vi "fft.vi"() -> ()   [LabVIEW 2013]
uses:
  <vilib>/ptbypt/Frequency Domain.llb/Real FFT PtByPt.vi
  <userlib>/_MGI/1D Array/MGI Running Average/MGI Running Average(DBL).vi
  <vilib>/Analysis/NI_AALBase.lvlib
  <vilib>/ptbypt/NI_PtbyPt.lvlib
panel:
  in  "Do Everything":bool
  out "maxima indexes":i32[](array[numeric])
  out "run ave check":bool
  out "Err Peak Cluster":dbl
  out "Err  Peak":dbl
  in  "stop":bool
  out "freqout Peak Cluster":dbl format="%#_10g"
  out "freqout Peak":dbl
  in  "Analyze FFT":bool
  out "FFT Graph":dbl[](graph)
  out "xscale multiplierNEW":dbl
  in  "#samples":i32=5000
  in  "Take FFT":bool
  out "Waveform Graph NEW":dbl[][](graph)
  in  "Ampl DC":dbl
  in  "Ampl Noise(stdev)":dbl
  in  "Ampl 4":dbl
  in  "Ampl 3":dbl
  in  "Ampl 2":dbl
  in  "Ampl 1":dbl
  in  "Freq 4":dbl
  in  "Freq 3":dbl
  in  "Freq 2":dbl
  in  "Freq 1":dbl
  in  "Active Noise":bool
  in  "Active 4":bool
  in  "Active 3":bool
  in  "Active 2":bool
  in  "Active 1":bool
  in  "Active DC":bool
  in  "fs":i32=10000
  in  "Build Waveform":bool
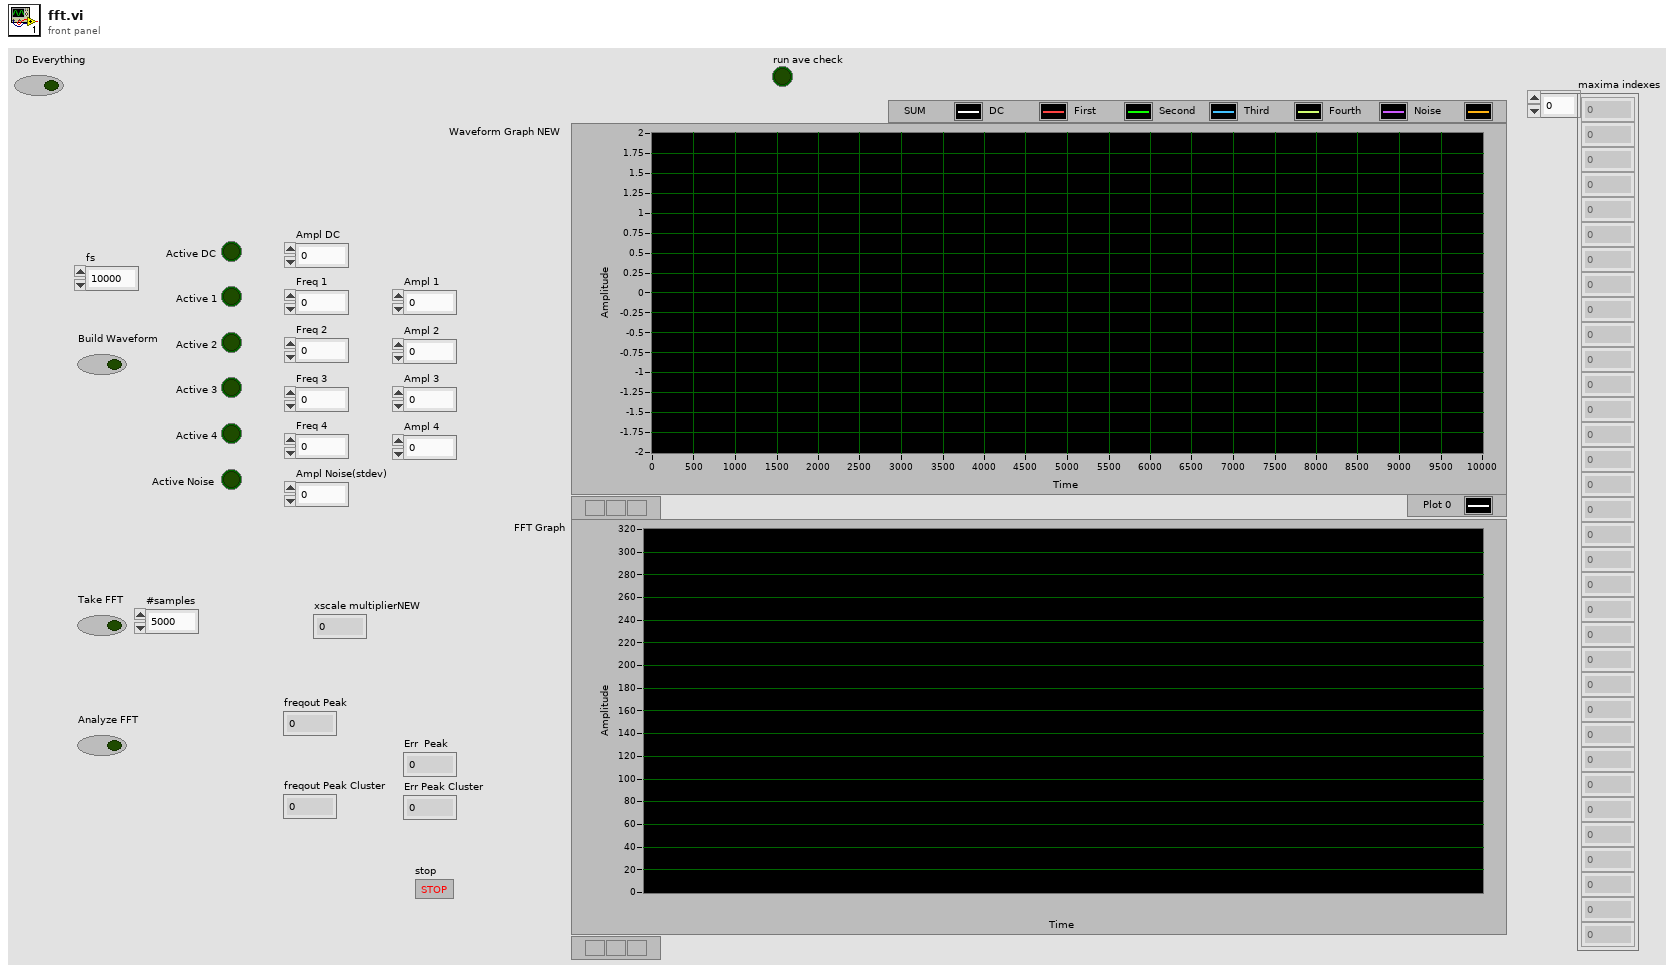
[diagram p1: front panel]
types:
  T1 = enum8{"Enabled", "Disabled", "Disabled and Grayed Out"}
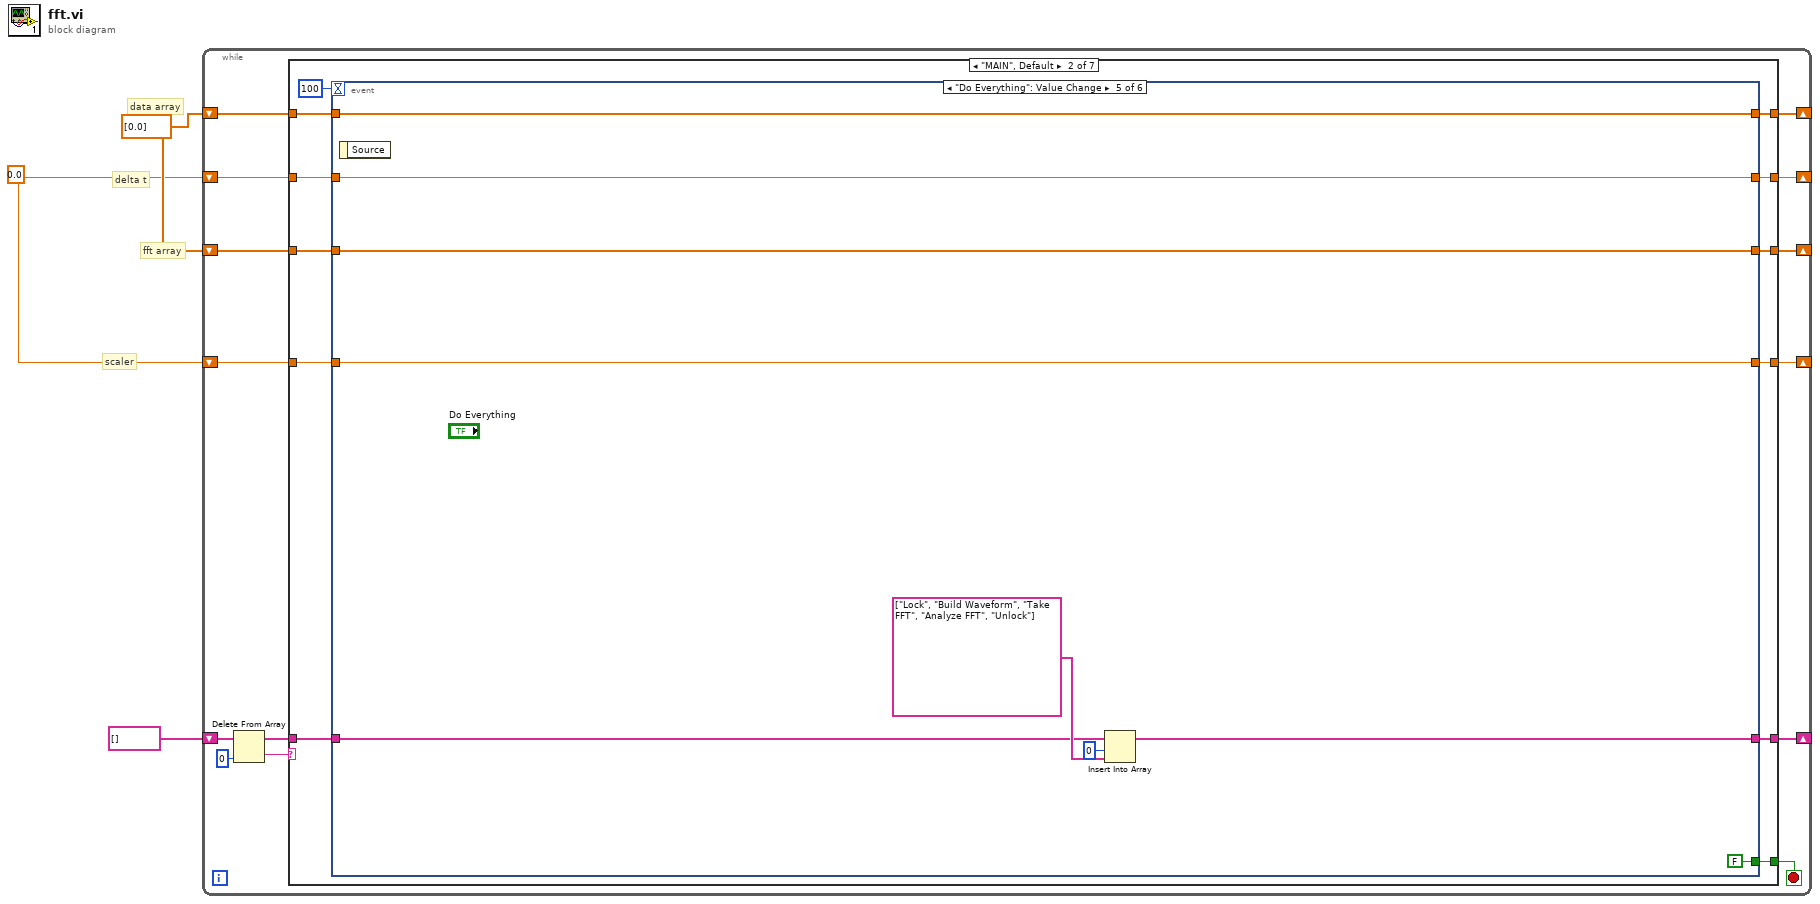
[diagram p0: block diagram]
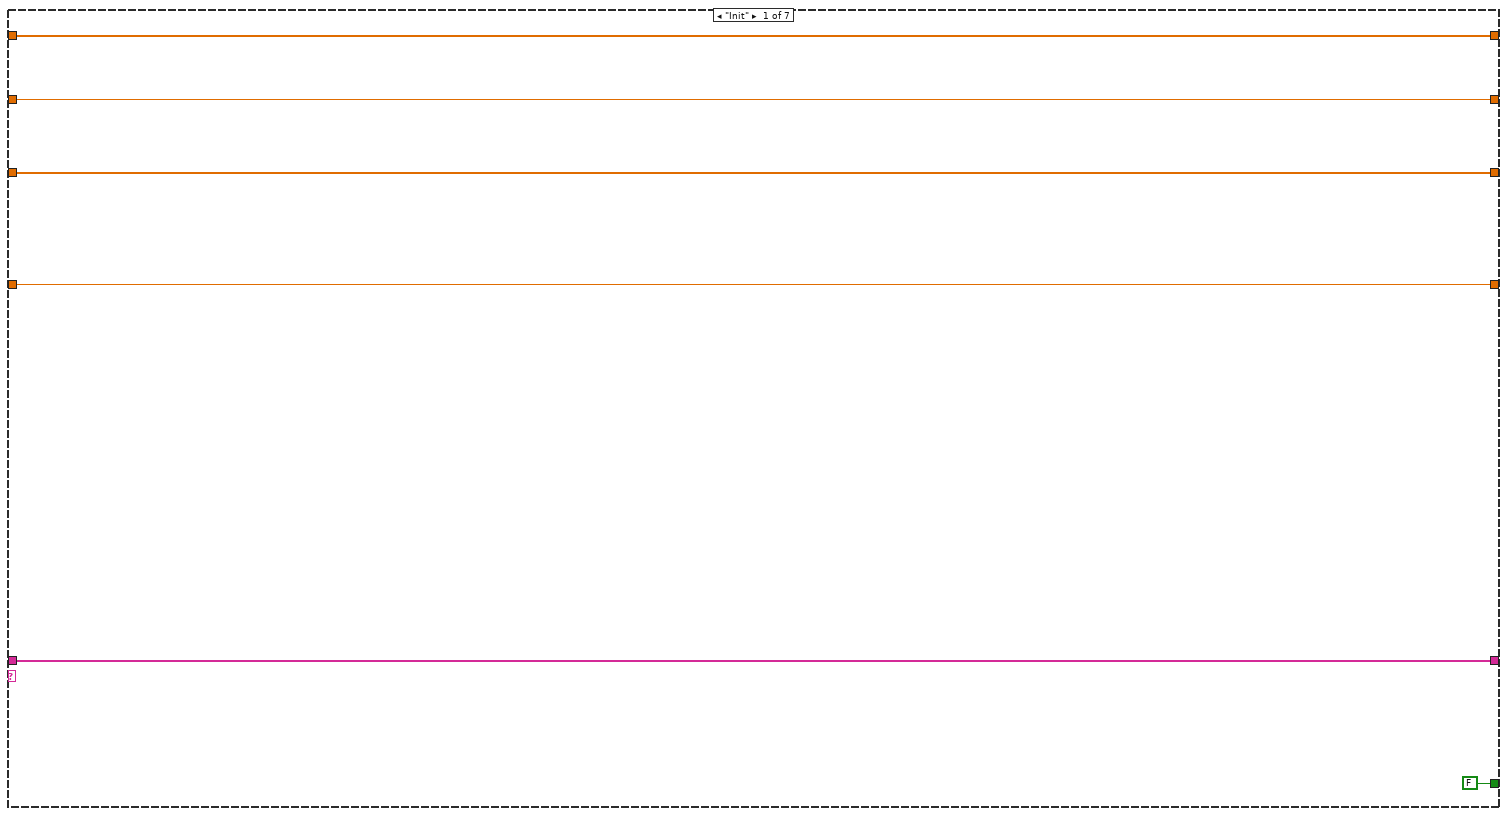
[diagram p2: hidden frame]
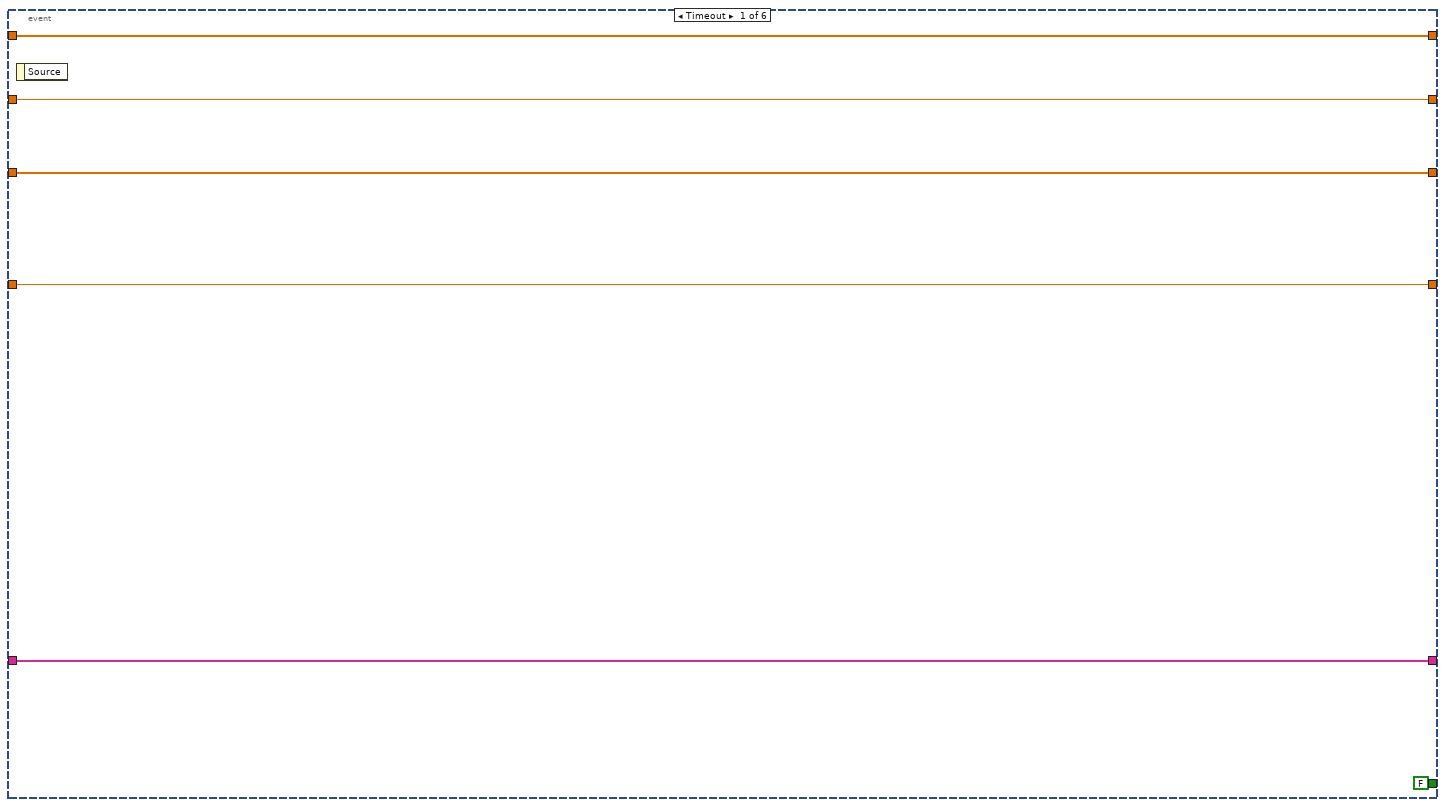
[diagram p3: hidden frame]
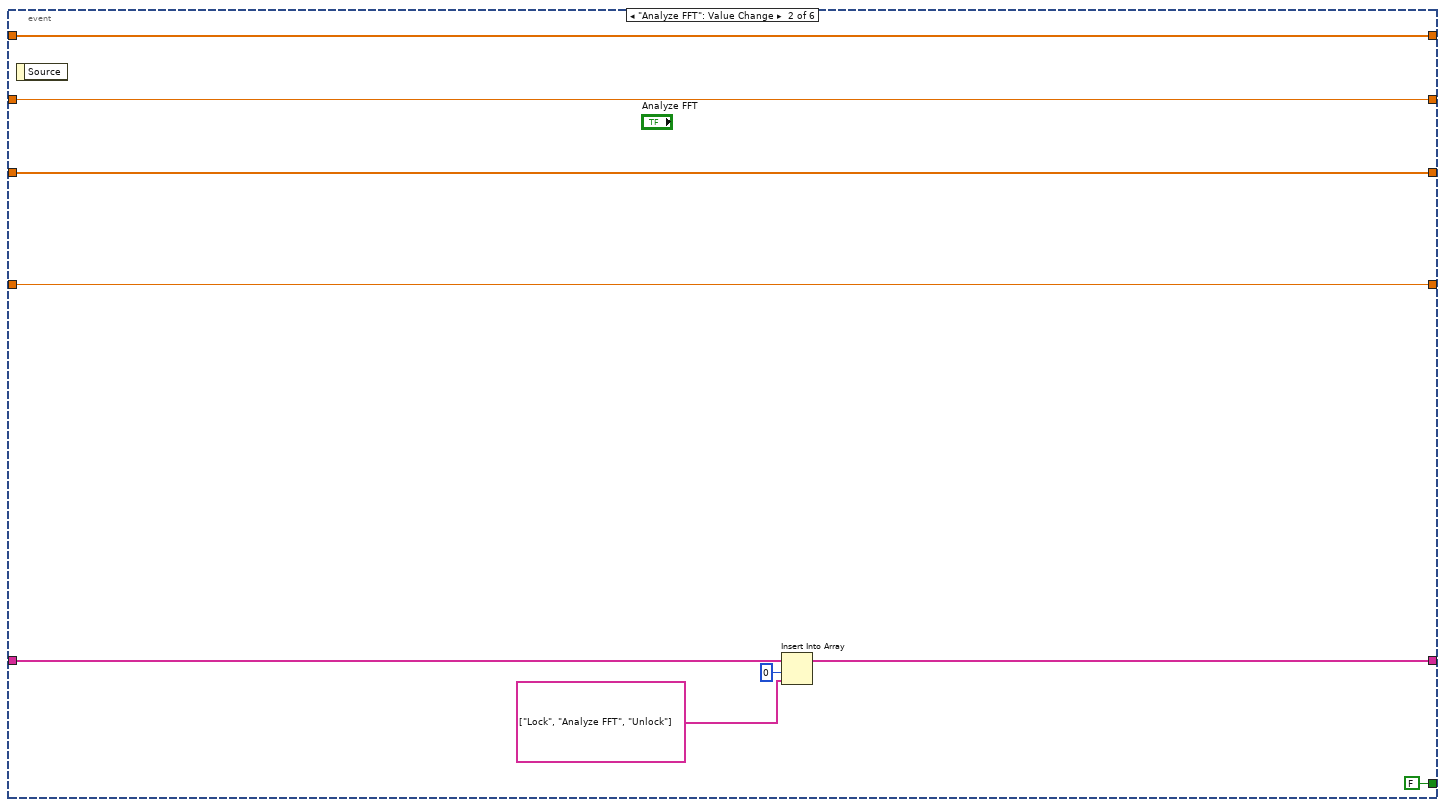
[diagram p4: hidden frame]
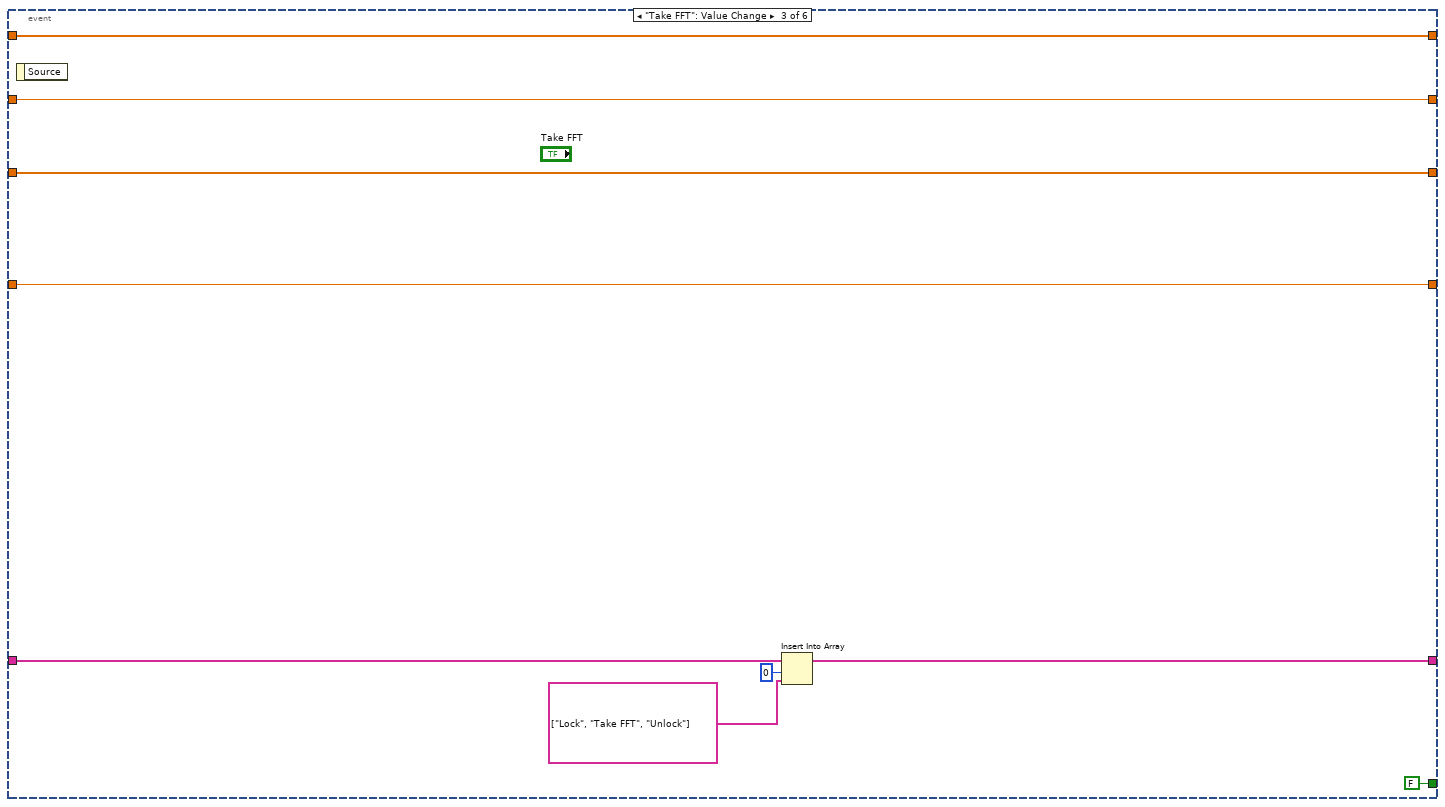
[diagram p5: hidden frame]
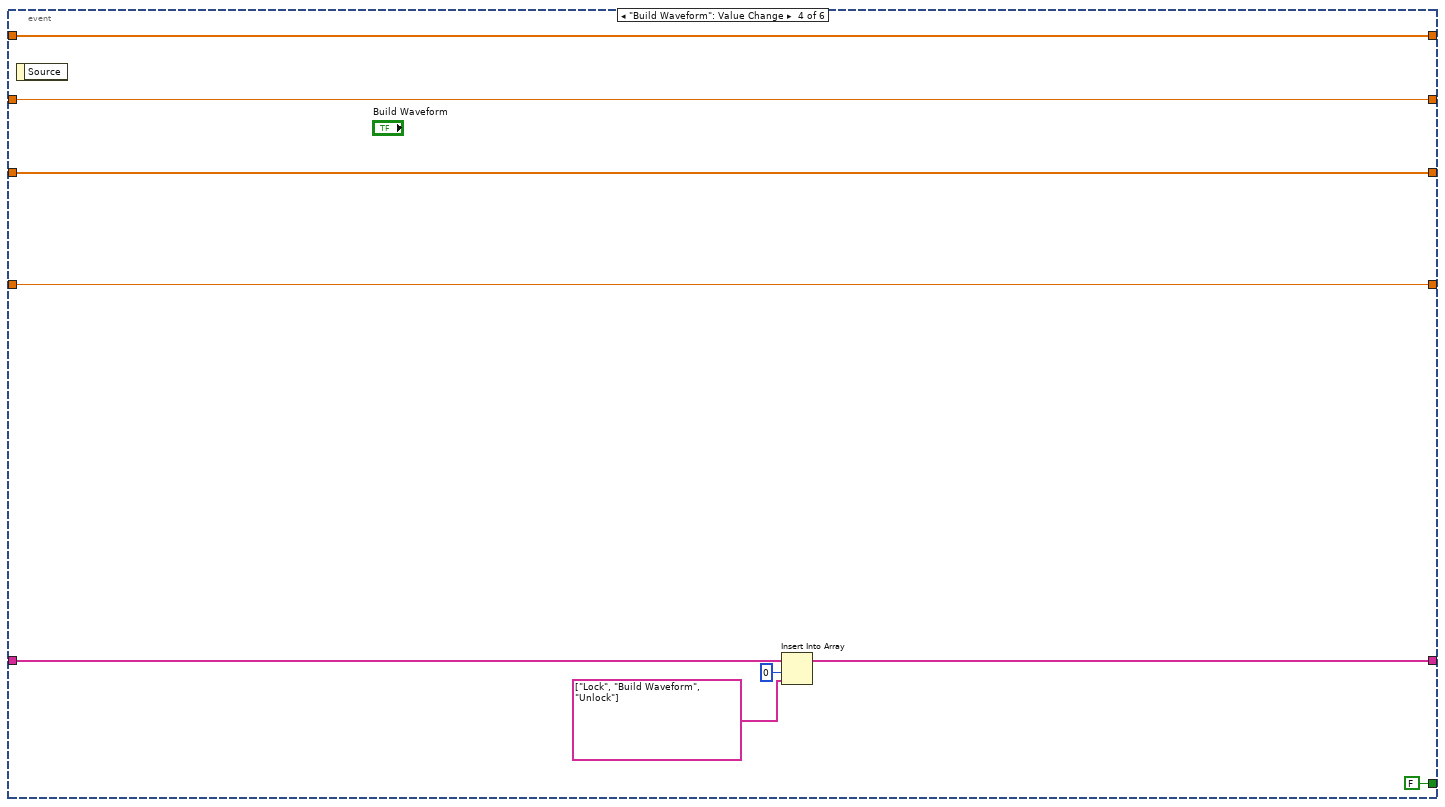
[diagram p6: hidden frame]
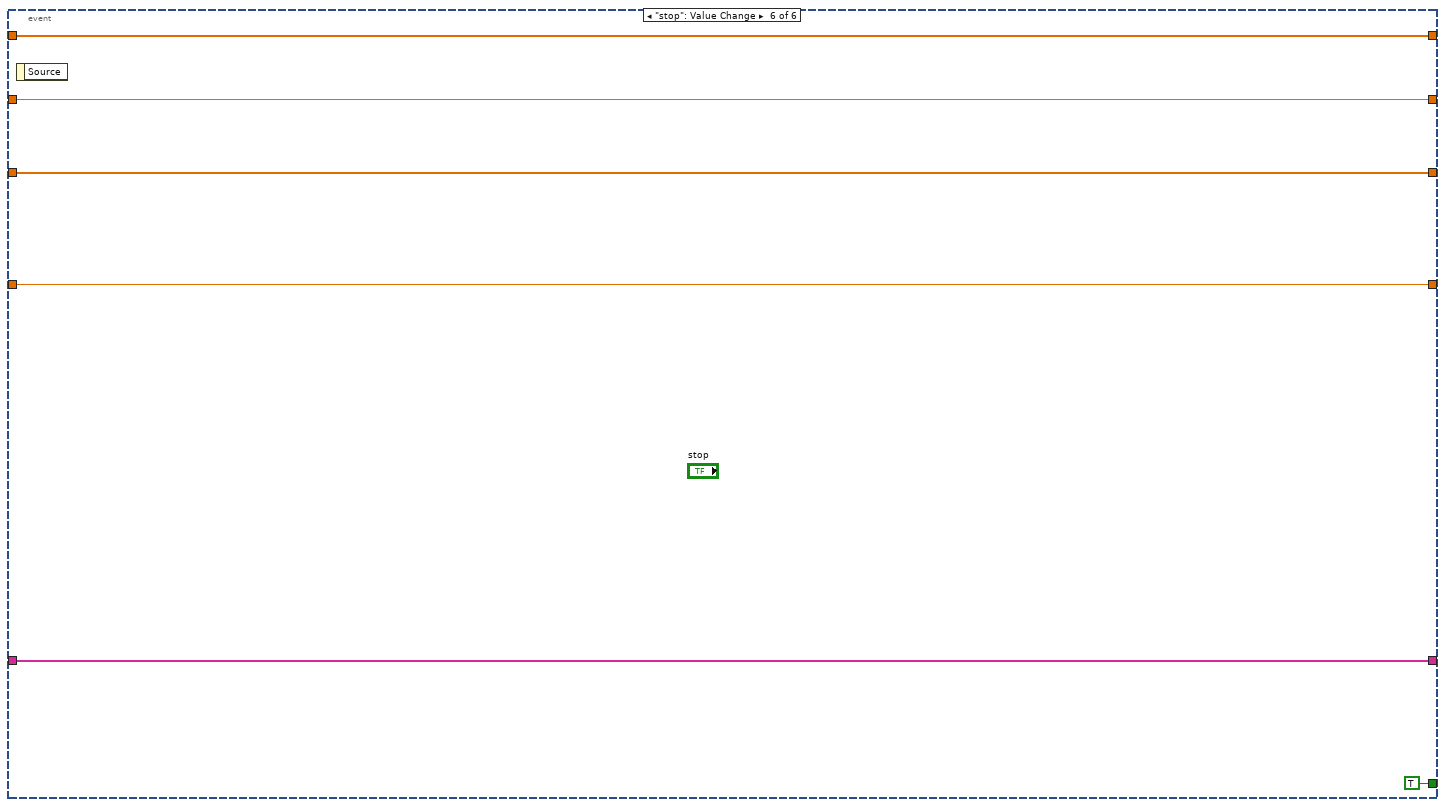
[diagram p7: hidden frame]
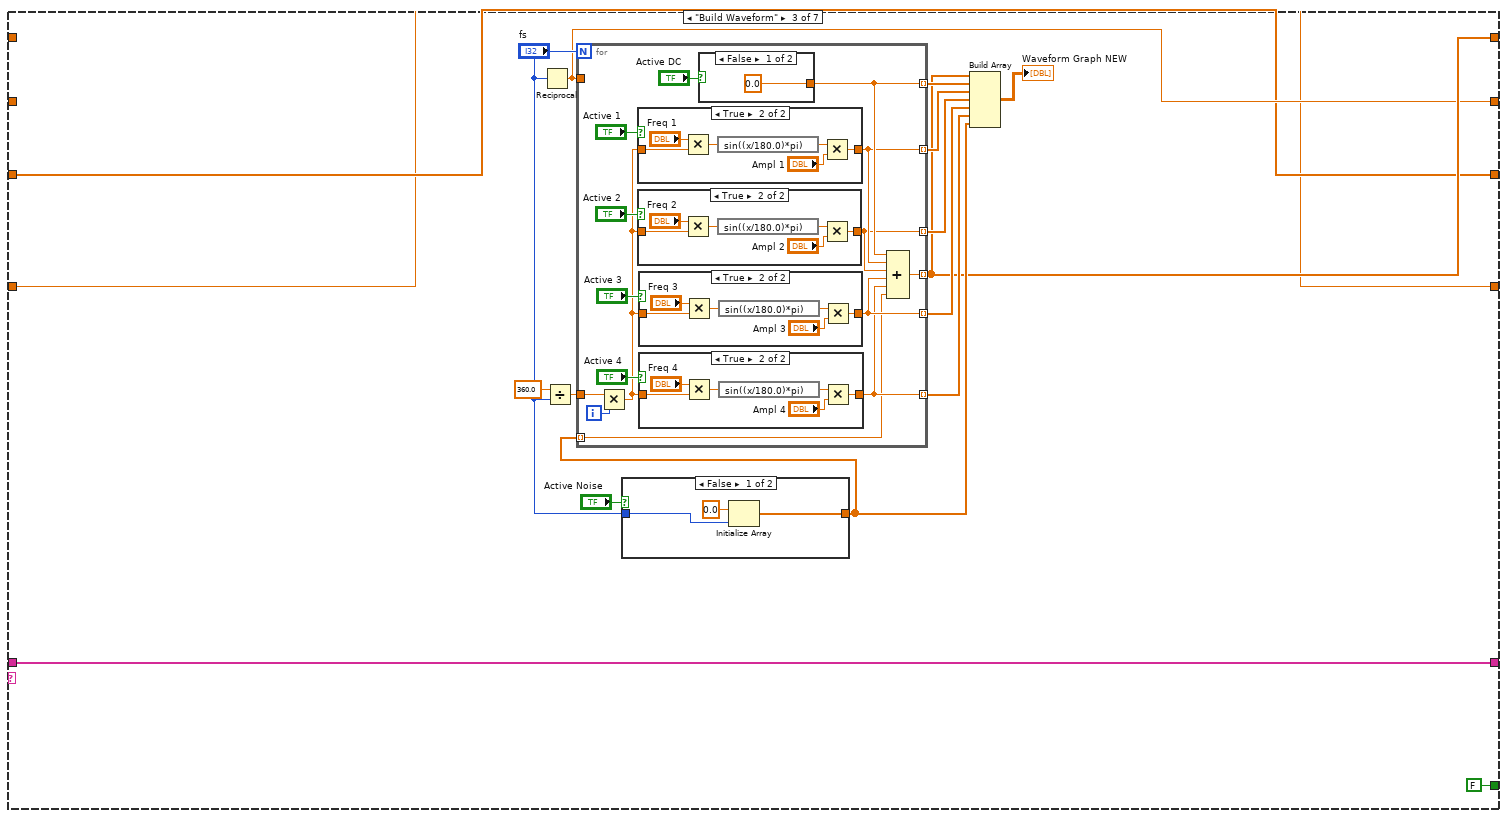
[diagram p8: hidden frame]
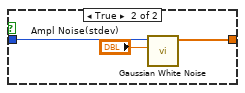
[diagram p9: hidden frame]
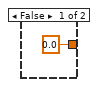
[diagram p10: hidden frame]
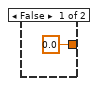
[diagram p11: hidden frame]
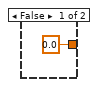
[diagram p12: hidden frame]
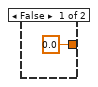
[diagram p13: hidden frame]
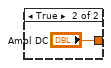
[diagram p14: hidden frame]
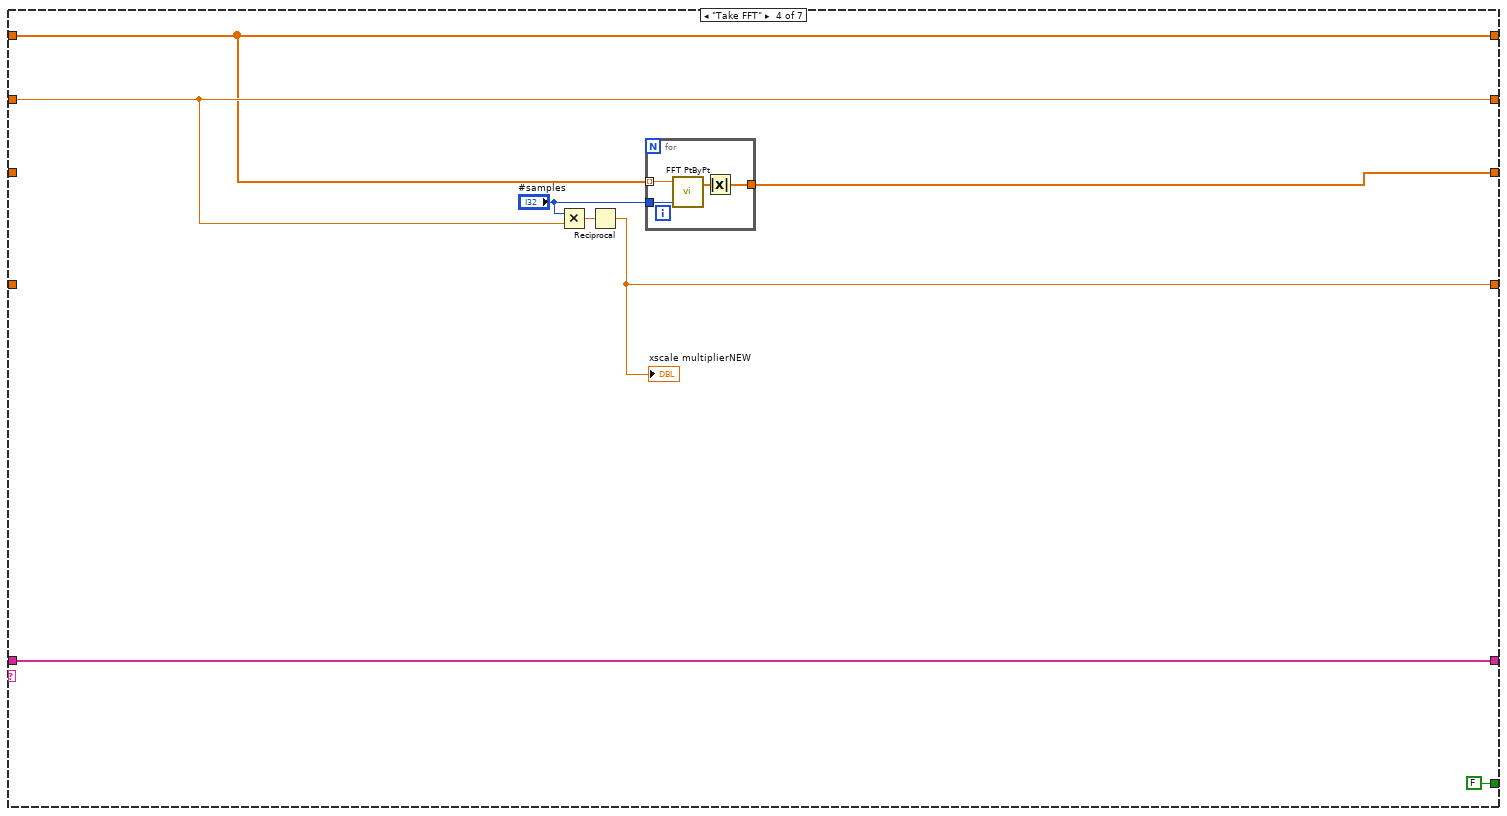
[diagram p15: hidden frame]
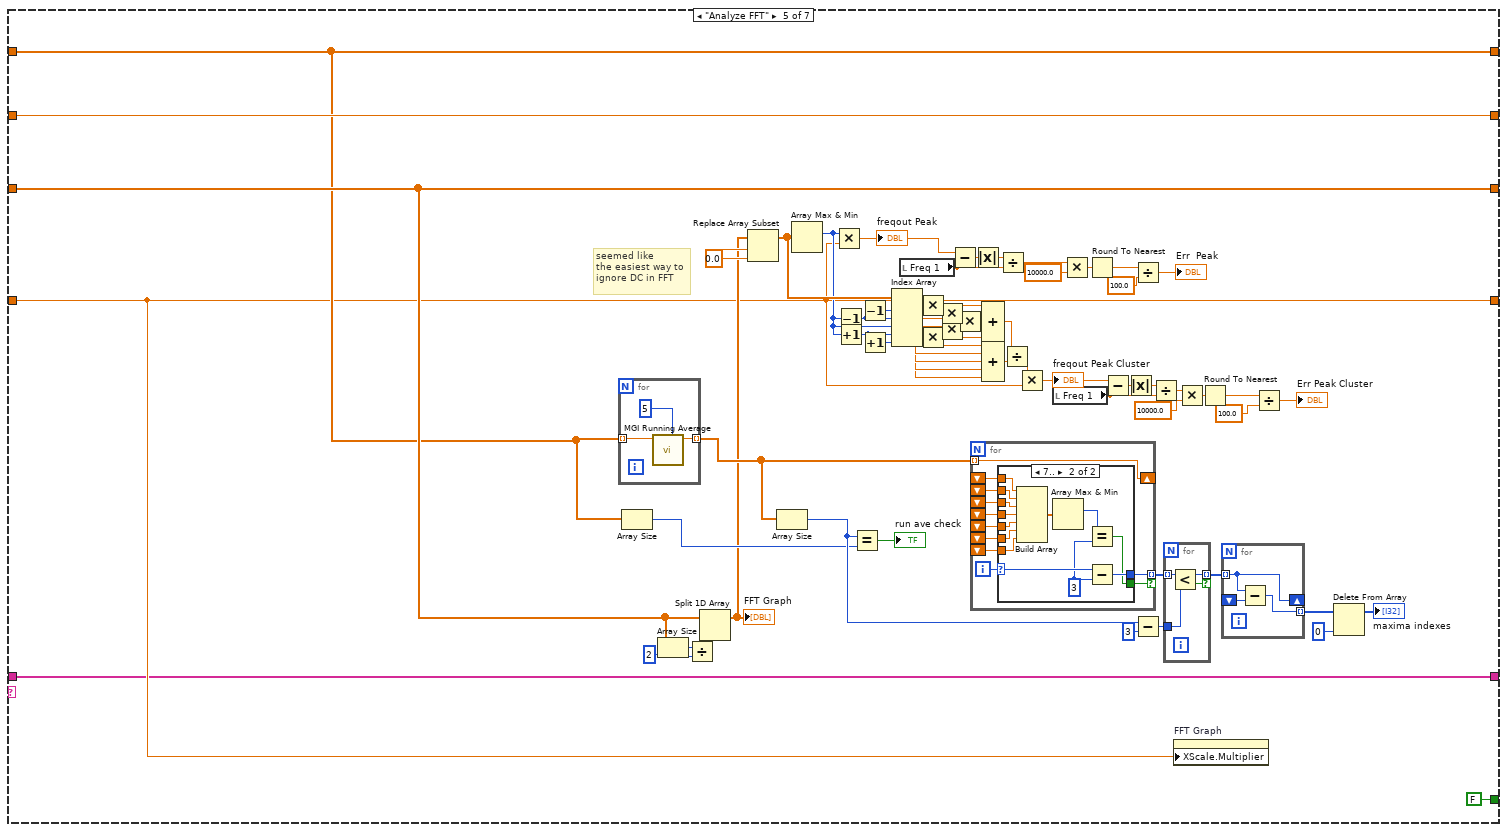
[diagram p16: hidden frame]
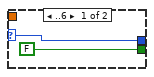
[diagram p17: hidden frame]
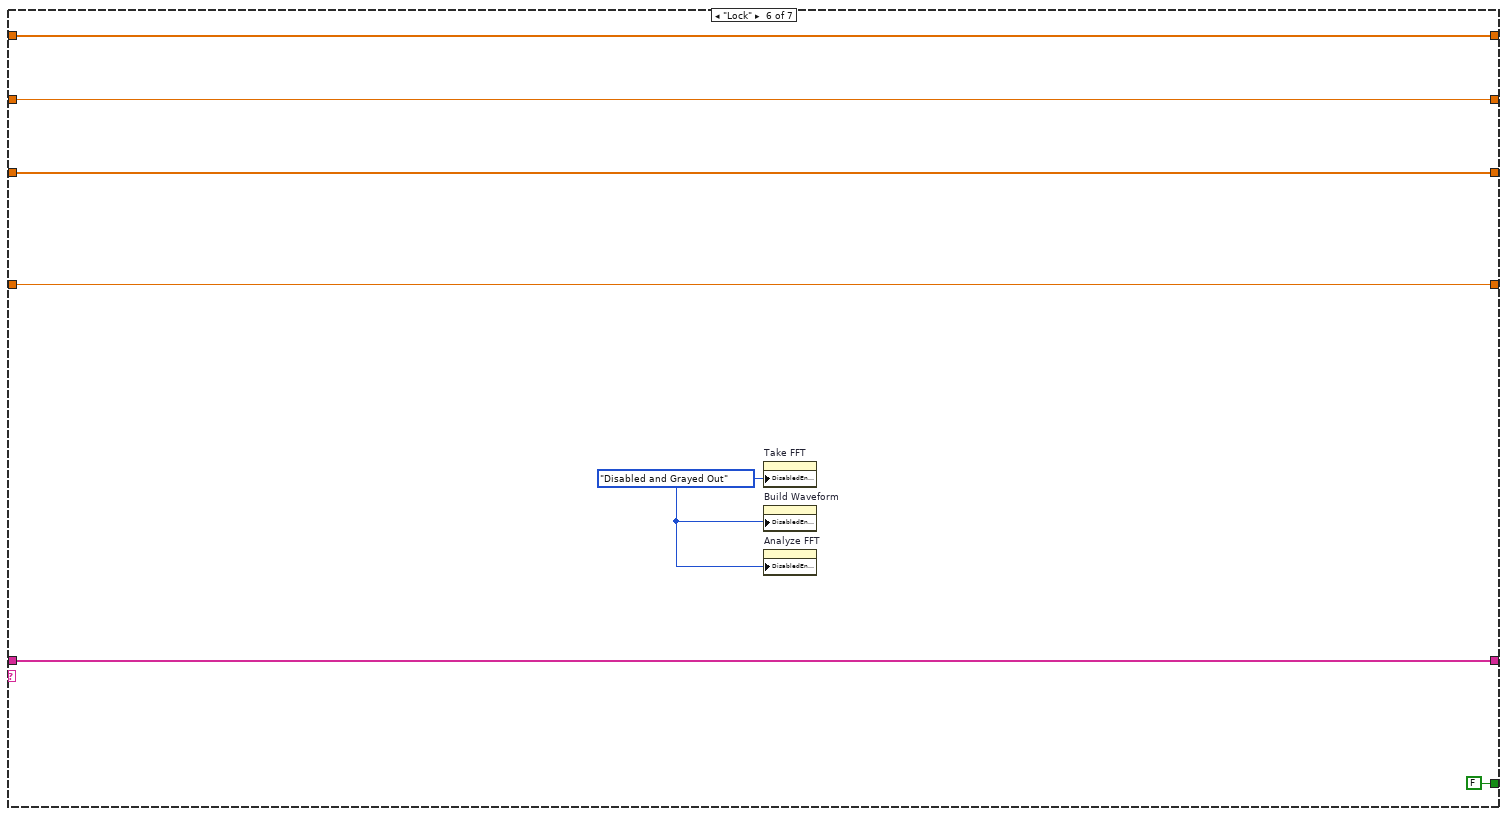
[diagram p18: hidden frame]
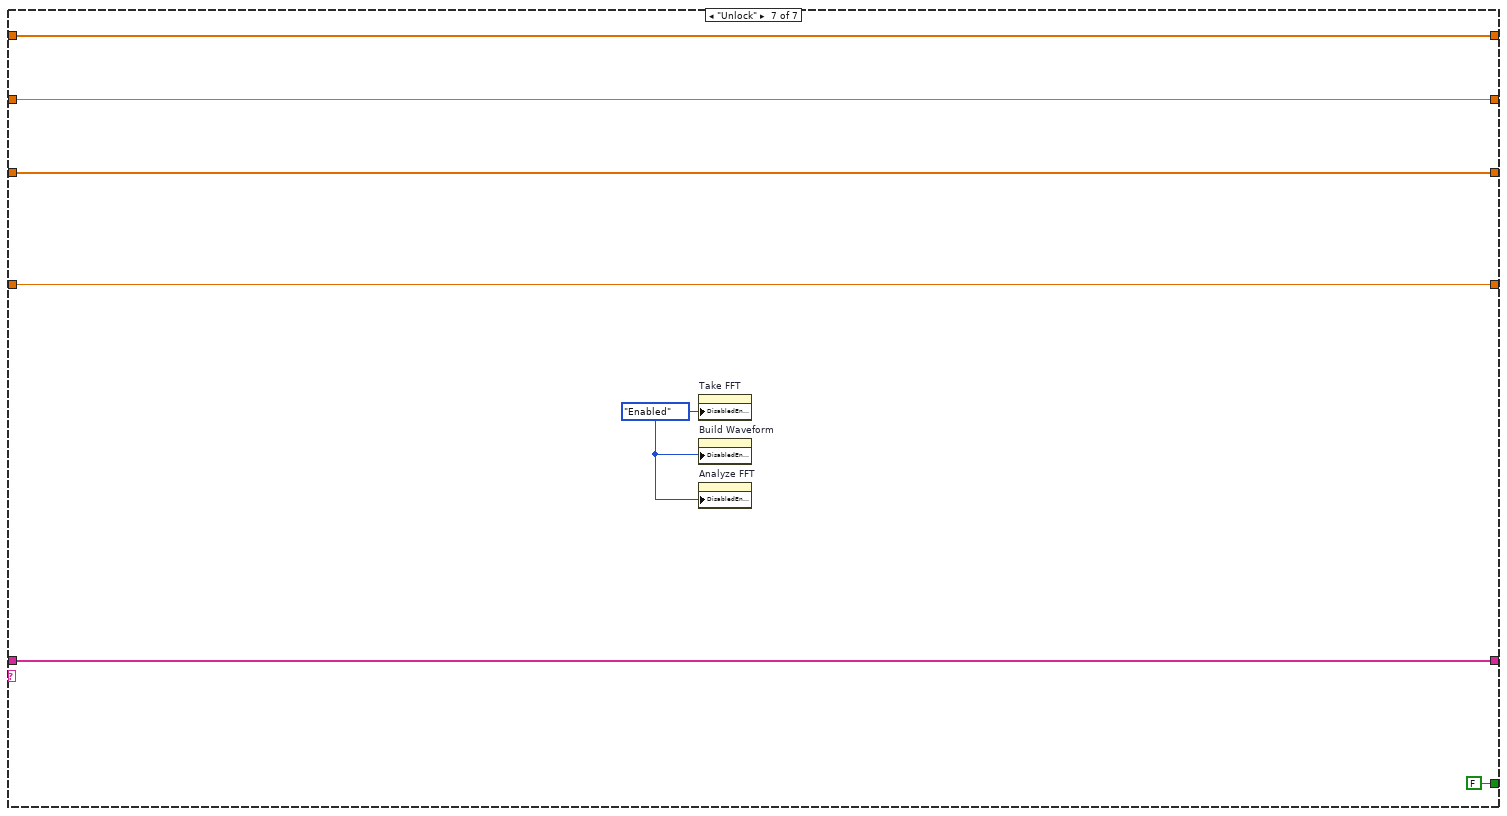
[diagram p19: hidden frame]
diagram:
  w1 = 0.0
  w2 = dbl[] [0.0]
  # "scaler"
  # "fft array"
  # "delta t"
  # "data array"
  n1 = while {
    shift-right: [w12] -> _
    shift-left: w2 -> [w13]
    shift-right: [w11] -> _
    shift-left: w1 -> [w10]
    shift-right: [w9] -> _
    shift-left: w2 -> [w8]
    shift-right: [w6] -> _
    shift-left: w1 -> [w7]
    shift-right: [w4] -> _
    shift-left: string[] [] -> [w17]
    stop <- w14 stop-if-true
    n2 = Delete From Array(array=w17, index=0) -> (deleted portion=w16:string, array with subset deleted=w5:string[])  [unwired: 1 in]
    n3 = case shown="\"MAIN\", Default" w16 {
      tunnel: [w23 w34 w87 w153 w165 w264 w269] -> w4
      tunnel: [FALSE w32 FALSE FALSE FALSE FALSE FALSE] -> w14
      tunnel: w13 -> [w21 w31 _ w156 w167 w260 w273]
      tunnel: [w21 w30 w89 w156 w167 w260 w273] -> w12
      tunnel: [w20 w28 w88 w157 w224 w261 w272] -> w11
      tunnel: w10 -> [w20 w29 _ w157 w224 w261 w272]
      tunnel: [w19 w26 w86 w155 w168 w262 w271] -> w9
      tunnel: w8 -> [w19 w27 w86 _ w168 w262 w271]
      tunnel: w7 -> [w18 w25 w85 _ w166 w263 w270]
      tunnel: [w18 w24 w85 w154 w166 w263 w270] -> w6
      tunnel: w5 -> [w23 w35 w87 w153 w165 w264 w269]
      frame "Init" {
      }
      frame "MAIN", Default {
        n4 = event shown="[4] \"Do Everything\": Value Change" {
          selector: _ -> [_ _ _ _ _ _]
          dyn-events: _ -> [_ _ _ _ _ _]
          timeout: 100 -> [_ _ _ _ _ _]
          tunnel: w35 -> [w41 w45 w52 w61 w71 w79]
          tunnel: [w41 w44 w51 w60 w70 w79] -> w34
          tunnel: [FALSE FALSE FALSE FALSE FALSE TRUE] -> w32
          tunnel: w31 -> [w39 w50 w59 w64 w77 w83]
          tunnel: [w39 w50 w59 w64 w77 w83] -> w30
          tunnel: w29 -> [w38 w49 w58 w65 w76 w82]
          tunnel: [w38 w49 w58 w65 w76 w82] -> w28
          tunnel: w27 -> [w37 w48 w57 w66 w75 w81]
          tunnel: [w37 w48 w57 w66 w75 w81] -> w26
          tunnel: w25 -> [w36 w47 w56 w67 w74 w80]
          tunnel: [w36 w47 w56 w67 w74 w80] -> w24
          event Timeout {
            n5 = event-data() -> ()  [unwired: 1 in, 1 out]
          }
          event "Analyze FFT": Value Change {
            n6 = event-data() -> ()  [unwired: 1 in, 1 out]
            n7 = Insert Into Array(array=w45, index=0, new element=string[] ["Lock", "Analyze FFT", "Unlock"]) -> (w44:string[])
          }
          event "Take FFT": Value Change {
            n8 = event-data() -> ()  [unwired: 1 in, 1 out]
            n9 = Insert Into Array(array=w52, index=0, new element=string[] ["Lock", "Take FFT", "Unlock"]) -> (w51:string[])
          }
          event "Build Waveform": Value Change {
            n10 = event-data() -> ()  [unwired: 1 in, 1 out]
            n11 = Insert Into Array(array=w61, index=0, new element=string[] ["Lock", "Build Waveform", "Unlock"]) -> (w60:string[])
          }
          event "Do Everything": Value Change {
            n12 = event-data() -> ()  [unwired: 1 in, 1 out]
            n13 = Insert Into Array(array=w71, index=0, new element=string[] ["Lock", "Build Waveform", "Take FFT", "Analyze FFT", "Unlock"]) -> (w70:string[])
          }
          event "stop": Value Change {
            n14 = event-data() -> ()  [unwired: 1 in, 1 out]
          }
        }
      }
      frame "Build Waveform" {
        n15 = Reciprocal(x="fs") -> (1/x=w88:dbl)
        n16 = Divide(x=360.0, y="fs") -> (x/y=w100:dbl)
        n17 = case shown="False" "Active Noise" {
          tunnel: "fs" -> [w103 w105]
          tunnel: [w101 w104] -> w98
          frame False {
            n18 = Initialize Array(0.0 ("element"), w103) -> (w101:dbl[])
          }
          frame True {
            n19 = call <vilib>:"Gaussian White Noise.vi"("standard deviation"="Ampl Noise(stdev)", "samples"=w105) -> ("Gaussian noise pattern"=w104:dbl[])  [unwired: 8 in, 1 out]
          }
        }
        n20 = for {
          N: "fs" -> [_]
          tunnel: w88 -> [_]
          tunnel: w100 -> [w121]
          tunnel: [w111] -> w95 mode=indexing
          tunnel: [w112] -> w94 mode=indexing
          tunnel: [w113] -> w93 mode=indexing
          tunnel: [w110] -> w96 mode=indexing
          tunnel: [w109] -> w97 mode=indexing
          tunnel: w98 -> [w108] mode=indexing
          tunnel: [w107] -> w89 mode=indexing
          i -> [w120]
          n21 = Multiply(x=w121, y=w120) -> (x*y=w114:dbl)
          n22 = case shown="True" "Active 1" {
            tunnel: [0.0 w145] -> w112
            tunnel: w114 -> [_ w144]
            frame False {
            }
            frame True {
              n23 = Multiply(x="Freq 1", y=w144) -> (x*y=w148:dbl)
              n24 = expression code="sin((x/180.0)*pi)"(w148) -> (w147:dbl)
              n25 = Multiply(x=w147, y="Ampl 1") -> (x*y=w145:dbl)
            }
          }
          n26 = case shown="True" "Active 2" {
            tunnel: [0.0 w138] -> w111
            tunnel: w114 -> [_ w137]
            frame False {
            }
            frame True {
              n27 = Multiply(x="Freq 2", y=w137) -> (x*y=w141:dbl)
              n28 = expression code="sin((x/180.0)*pi)"(w141) -> (w140:dbl)
              n29 = Multiply(x=w140, y="Ampl 2") -> (x*y=w138:dbl)
            }
          }
          n30 = case shown="True" "Active 3" {
            tunnel: [0.0 w131] -> w110
            tunnel: w114 -> [_ w130]
            frame False {
            }
            frame True {
              n31 = Multiply(x="Freq 3", y=w130) -> (x*y=w134:dbl)
              n32 = expression code="sin((x/180.0)*pi)"(w134) -> (w133:dbl)
              n33 = Multiply(x=w133, y="Ampl 3") -> (x*y=w131:dbl)
            }
          }
          n34 = case shown="True" "Active 4" {
            tunnel: [0.0 w124] -> w109
            tunnel: w114 -> [_ w123]
            frame False {
            }
            frame True {
              n35 = Multiply(x="Freq 4", y=w123) -> (x*y=w127:dbl)
              n36 = expression code="sin((x/180.0)*pi)"(w127) -> (w126:dbl)
              n37 = Multiply(x=w126, y="Ampl 4") -> (x*y=w124:dbl)
            }
          }
          n38 = case shown="False" "Active DC" {
            tunnel: [0.0 ("Ampl DC") "Ampl DC"] -> w113
            frame False {
            }
            frame True {
            }
          }
          n39 = Compound Arithmetic op=ADD(w113, w112, w111, w110, w109, w108) -> (w107:dbl)
        }
        n40 = Build Array(w89, w93, w94, w95, w96, w97, w98) -> (→"Waveform Graph NEW":dbl[][])
      }
      frame "Take FFT" {
        n41 = Multiply(x="#samples", y=w157) -> (x*y=w158:dbl)
        n42 = Reciprocal(x=w158) -> (1/x=w154:dbl)
        "xscale multiplierNEW" <- w154
        n43 = for {
          tunnel: w156 -> [w163] mode=indexing
          tunnel: "#samples" -> [w162]
          tunnel: [w160] -> w155
          n44 = call-poly <vilib>:"FFT PtByPt.vi"("sample length"=w162, "x"=w163) -> ("FFT{X}"=w161:cdb[])  [unwired: 2 in, 1 out]
          n45 = Absolute Value(x=w161) -> (abs(x)=w160:dbl[])
        }
      }
      frame "Analyze FFT" {
        w212 = 0.0 ("new element/subarray")
        # "seemed like\nthe easiest way to\nignore DC in FFT"
        n46 = for {
          tunnel: w167 -> [w226] mode=indexing
          tunnel: [w225] -> w214 mode=indexing
          n47 = call-poly <userlib>:"MGI Running Average.vi"("Averaging Size"=5, "Value"=w226) -> ("Average"=w225:dbl)  [unwired: 9 in]
        }
        n48 = Array Size(array=w167) -> (size(s)=w213:i32)
        n49 = Array Size(array=w168) -> (size(s)=w170:i32)
        n50 = Divide(x=w170, y=2) -> (x/y=w169:dbl)
        n51 = Split 1D Array(array=w168, index=w169) -> (first subarray=w210:dbl[])  [unwired: 1 out]
        "FFT Graph" <- w210
        n52 = Replace Array Subset(array=w210, new element=w212, index=w212) -> (w211:dbl[])
        n53 = Array Size(array=w214) -> (size(s)=w217:i32)
        n54 = Array Max & Min(array=w211) -> (max index (indices)=w174:i32)  [unwired: 3 out]
        n55 = Multiply(x=w174, y=w166) -> (x*y=w193:dbl)
        "freqout Peak" <- w193
        n56 = Decrement(x=w174) -> (x-1=w175:i32)
        n57 = Increment(x=w174) -> (x+1=w173:i32)
        n58 = Equal?(x=w217, y=w213) -> (x = y?=→"run ave check":bool)
        n59 = Decrement(x=w175) -> (x-1=w176:i32)
        n60 = Increment(x=w173) -> (x+1=w172:i32)
        n61 = Index Array(array=w211, index #1=w176, index #2=w175, index #3=w174, index #4=w173, index #5=w172) -> (element #1=w189:dbl, element #2=w188:dbl, element #3=w187:dbl, element #4=w186:dbl, element #5=w185:dbl)
        n62 = local read "Freq 1"() -> (w192:dbl)
        n63 = Multiply(x=w176, y=w189) -> (x*y=w177:dbl)
        n64 = Multiply(x=w172, y=w185) -> (x*y=w181:dbl)
        n65 = Multiply(x=w175, y=w188) -> (x*y=w178:dbl)
        n66 = Multiply(x=w173, y=w186) -> (x*y=w180:dbl)
        n67 = Subtract(x=w193, y=w192) -> (x-y=w190:dbl)
        n68 = Multiply(x=w174, y=w187) -> (x*y=w179:dbl)
        n69 = for {
          tunnel: w214 -> [w244] mode=indexing
          shift-right: [w244] -> _
          shift-left: _ -> [w242]
          shift-left: _ -> [w241]
          shift-left: _ -> [w240]
          shift-left: _ -> [w239]
          shift-left: _ -> [w238]
          shift-left: _ -> [w237]
          shift-left: _ -> [w236]
          tunnel: [w235] -> w216 mode=indexing if=w234
          i -> [w243]
          n70 = case shown="7.." w243 {
            selector: w243 -> [w246 w259]
            tunnel: w242 -> [_ w258]
            tunnel: w241 -> [_ w257]
            tunnel: w240 -> [_ w256]
            tunnel: w239 -> [_ w255]
            tunnel: w238 -> [_ w254]
            tunnel: w237 -> [_ w253]
            tunnel: w236 -> [_ w252]
            tunnel: [w246 w248] -> w235
            tunnel: [FALSE w247] -> w234
            frame ..6 {
            }
            frame 7.. {
              w249 = 3 ("y")
              n71 = Build Array(w258, w257, w256, w255, w254, w253, w252) -> (w251:dbl[])
              n72 = Array Max & Min(array=w251) -> (max index (indices)=w250:i32)  [unwired: 3 out]
              n73 = Equal?(x=w250, y=w249) -> (x = y?=w247:bool)
              n74 = Subtract(x=w259, y=w249) -> (x-y=w248:i32)
            }
          }
        }
        n75 = Absolute Value(x=w190) -> (abs(x)=w191:dbl)
        n76 = Compound Arithmetic op=ADD(w177, w178, w179, w180, w181) -> (w182:dbl)
        n77 = Compound Arithmetic op=ADD(w189, w188, w187, w186, w185) -> (w183:dbl)
        n78 = Divide(x=w191, y=w192) -> (x/y=w200:dbl)
        n79 = Divide(x=w182, y=w183) -> (x/y=w184:dbl)
        n80 = Multiply(x=w184, y=w166) -> (x*y=w197:dbl)
        "freqout Peak Cluster" <- w197
        n81 = local read "Freq 1"() -> (w194:dbl)
        n82 = Multiply(x=w200, y=10000.0) -> (x*y=w202:dbl)
        n83 = Round To Nearest(number=w202) -> (nearest integer value=w205:dbl)
        n84 = Subtract(x=w197, y=w194) -> (x-y=w196:dbl)
        n85 = Absolute Value(x=w196) -> (abs(x)=w195:dbl)
        n86 = Divide(x=w205, y=100.0) -> (x/y=→"Err  Peak":dbl)
        n87 = Subtract(x=w217, y=3) -> (x-y=w219:i32)
        n88 = Divide(x=w195, y=w194) -> (x/y=w201:dbl)
        n89 = for {
          tunnel: w216 -> [w232] mode=indexing
          tunnel: w219 -> [w233]
          tunnel: [w232] -> w220 mode=indexing if=w231
          n90 = Less?(x=w232, y=w233) -> (x < y?=w231:bool)
        }
        n91 = property on="FFT Graph" class="WFGraph (strict)"("XScale.Multiplier"=w166) -> ()  [unwired: 2 in, 2 out]
        n92 = Multiply(x=w201, y=10000.0) -> (x*y=w203:dbl)
        n93 = Round To Nearest(number=w203) -> (nearest integer value=w204:dbl)
        n94 = for {
          tunnel: w220 -> [w230] mode=indexing
          shift-right: [w230] -> _
          shift-left: _ -> [w229]
          tunnel: [w228] -> w221 mode=indexing
          n95 = Subtract(x=w230, y=w229) -> (x-y=w228:i32)
        }
        n96 = Divide(x=w204, y=100.0) -> (x/y=→"Err Peak Cluster":dbl)
        n97 = Delete From Array(array=w221, index=0) -> (array with subset deleted=→"maxima indexes":i32[])  [unwired: 1 in, 1 out]
      }
      frame "Lock" {
        w266 = T1."Disabled and Grayed Out" ("Disabled")
        n98 = property on="Take FFT" class="Bool"("DisabledEnum"=w266) -> ()  [unwired: 2 in, 2 out]
        n99 = property on="Build Waveform" class="Bool"("DisabledEnum"=w266) -> ()  [unwired: 2 in, 2 out]
        n100 = property on="Analyze FFT" class="Bool"("DisabledEnum"=w266) -> ()  [unwired: 2 in, 2 out]
      }
      frame "Unlock" {
        w267 = T1."Enabled" ("Disabled")
        n101 = property on="Take FFT" class="Bool"("DisabledEnum"=w267) -> ()  [unwired: 2 in, 2 out]
        n102 = property on="Build Waveform" class="Bool"("DisabledEnum"=w267) -> ()  [unwired: 2 in, 2 out]
        n103 = property on="Analyze FFT" class="Bool"("DisabledEnum"=w267) -> ()  [unwired: 2 in, 2 out]
      }
    }
  }
